vi "2D data.vi"() -> ()   [LabVIEW 2019]
panel:
  out "sorted array":T1(array[cluster])
  out "Array":T1(array[cluster])
  in  "dt 2":u32
  out "XY Graph 3":cluster{"X":dbl, "Y":dbl}[](graph)
  out "Waveform Graph 2":dbl[](graph)
  out "XY Graph 2":cluster{"X":dbl, "Y":dbl}[](graph)
  in  "dt":u32
  in  "index":i32
  in  "stop":bool
  out "XY Graph":cluster{"X":dbl, "Y":dbl}[](graph)
  out "Array 3":cluster{"Array":cluster{"x":dbl, "y":dbl}[]}[](array[cluster])
  out "Array 2":cluster{"x":dbl, "y":dbl}[](array[cluster]) {"x" format="%.3f"; "y" format="%.3f"}
  in  "limit_ptn":dbl
  in  "limit_len":dbl
  out "Waveform Graph":dbl[](graph)
  out "XY 그래프":cluster{"X":dbl, "Y":dbl}[](graph)
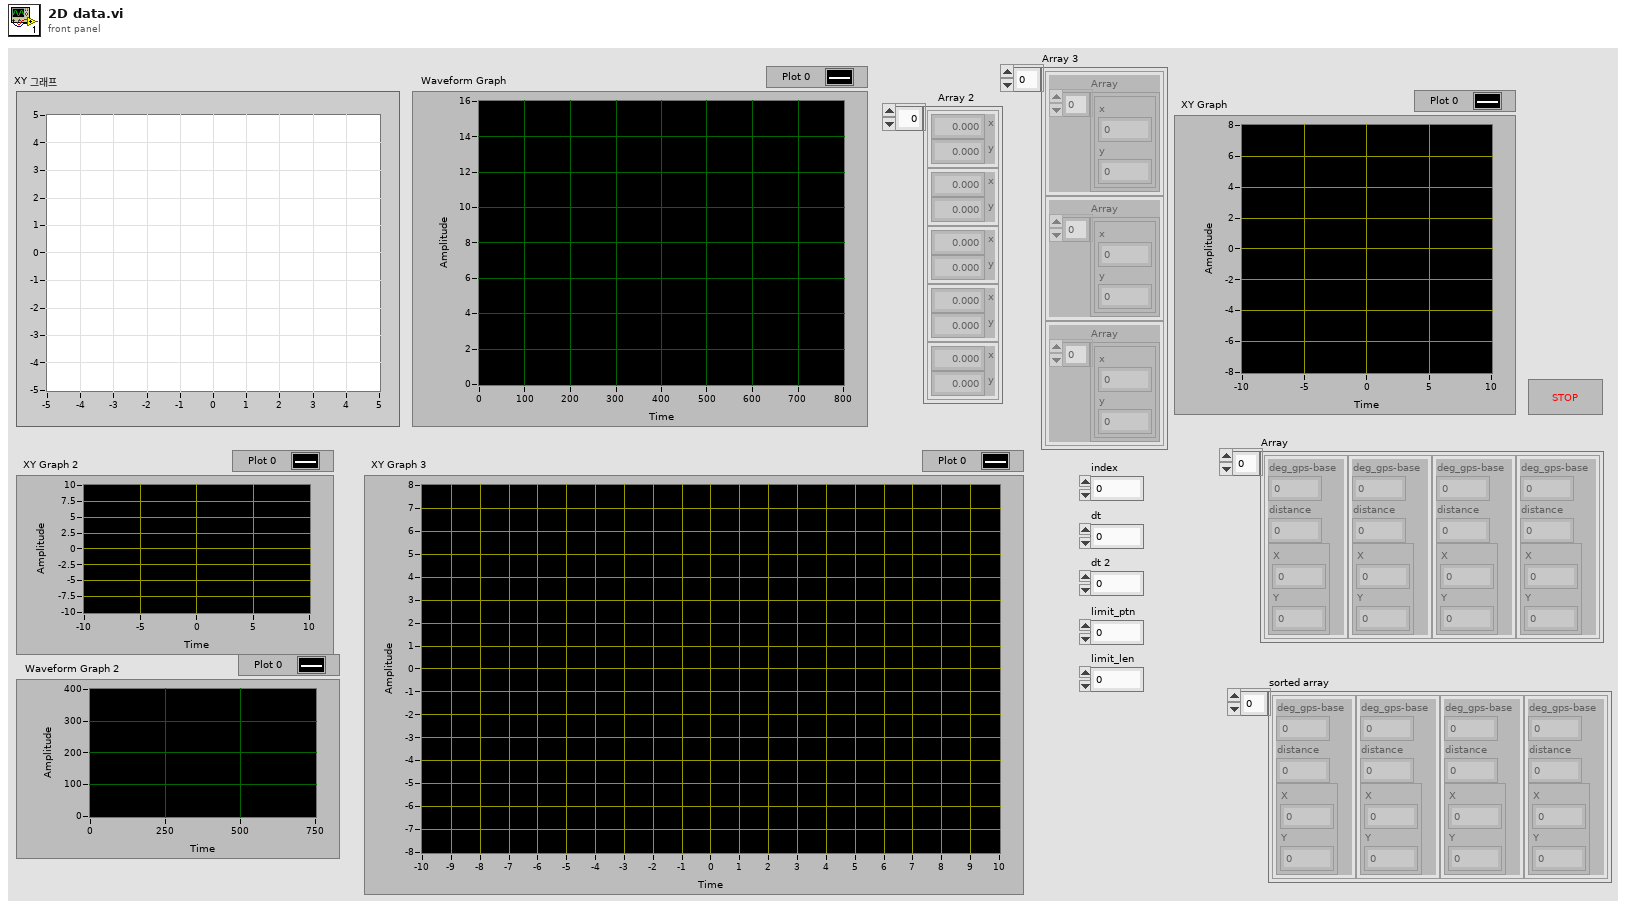
[diagram p1: front panel]
types:
  T1 = cluster{"deg_gps-base":dbl, "distance":dbl, cluster{"X":dbl, "Y":dbl}}[]
  T2 = cluster{"deg_gps-base":dbl, "distance":dbl, "xy":cluster{"X":dbl, "Y":dbl}}
  T3 = cluster{"deg_gps-base":dbl, "distance":dbl, "xy":cluster{"X":dbl, "Y":dbl}}[]
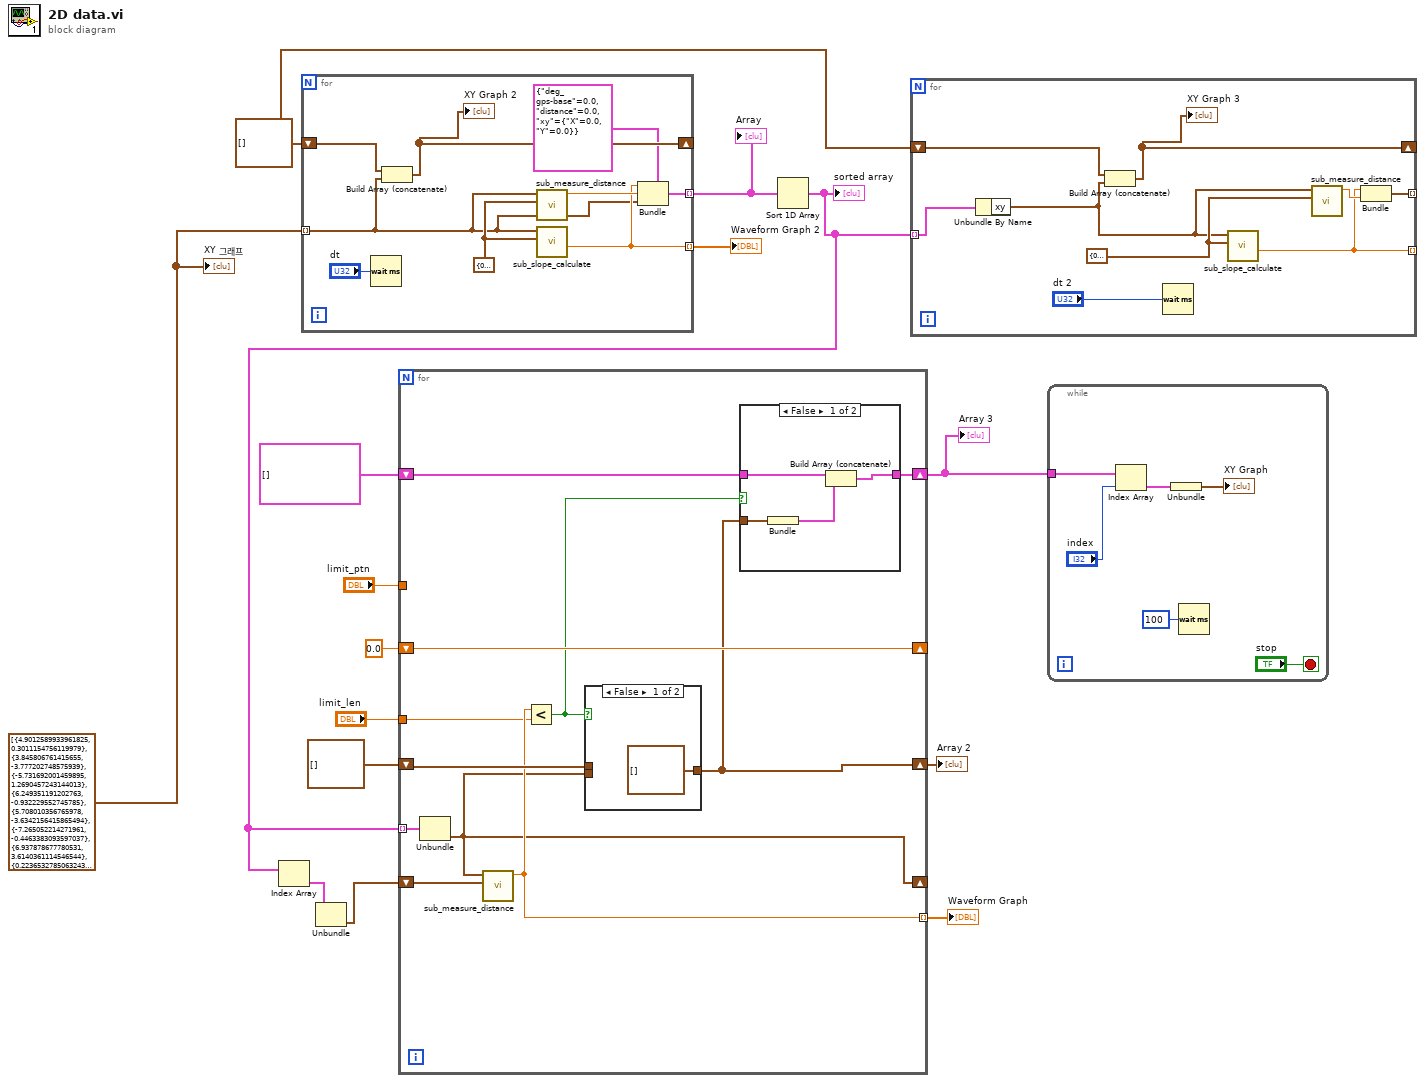
[diagram p0: block diagram]
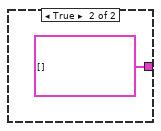
[diagram p2: hidden frame]
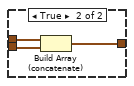
[diagram p3: hidden frame]
diagram:
  w4 = cluster{"X":dbl, "Y":dbl}[] []
  w7 = cluster{"X":dbl, "Y":dbl}[] [{"X"=4.9012589933961825, "Y"=0.3011154756119979}, {"X"=3.845806761415655, "Y"=-3.777202748575939}, {"X"=-5.731692001459895, "Y"=1.2690457243144013}, {"X"=6.249351191202763, "Y"=-0.932229552745785}, {"X"=5.708010356765978, "Y"=-3.6342156415865494}, {"X"=-7.265052214271961, "Y"=-0.4463383093597037}, {"X"=6.937878677780531, "Y"=3.6140361114546544}, {"X"=0.2236532785063243, "Y"=-0.08355102341307699}, {"X"=-0.27698848468565956, "Y"=-0.16663715627537012}, {"X"=-0.2822133509219429, "Y"=-0.16468511487504972}, {"X"=-0.2859435267244487, "Y"=-0.1632233501199644}, {"X"=-0.28971777798992493, "Y"=-0.16059318670659908}, {"X"=-0.2940448834529576, "Y"=-0.15840961623315852}, {"X"=-0.29848859861914145, "Y"=-0.15590099099871388}, {"X"=-0.3029295017509801, "Y"=-0.15383035938625036}, {"X"=-0.30807578671647845, "Y"=-0.15192616509022697}, {"X"=-0.31198972851346785, "Y"=-0.15017147466177655}, {"X"=-0.3163416286007537, "Y"=-0.14740751003331817}, {"X"=-0.32101017207613314, "Y"=-0.14502596982489518}, {"X"=-0.3256611193653853, "Y"=-0.14318832994935127}, {"X"=-0.33034585271792694, "Y"=-0.14118137303506342}, {"X"=-0.3370576037947027, "Y"=-0.1387530962687796}, {"X"=-0.34264737327116335, "Y"=-0.13626936592782707}, {"X"=-0.3452073355688534, "Y"=-0.13316116351794555}, {"X"=-0.34984706268427646, "Y"=-0.13080245690041115}, {"X"=-0.35583414812945, "Y"=-0.1275384609636978}, {"X"=-0.3600731071546751, "Y"=-0.12453255600034033}, {"X"=-0.001185404569007749, "Y"=-0.0003966308205063658}, {"X"=-0.37126244120133567, "Y"=-0.10002224629163652}, {"X"=-0.3684838809764134, "Y"=-0.09486769450429589}, {"X"=-0.36852848189245996, "Y"=-0.08953949147744147}, {"X"=-0.3669884185966218, "Y"=-0.08409370140474674}, {"X"=-0.3637742793807322, "Y"=-0.0789831384602372}, {"X"=-0.3613291353197761, "Y"=-0.07484821954504285}, {"X"=-0.36027625980387135, "Y"=-0.06992865379608967}, {"X"=-0.44303585980691584, "Y"=-0.051334461379728295}, {"X"=-0.43939260085108517, "Y"=-0.04557636248450506}, {"X"=-0.43576159671713005, "Y"=-0.038962556724851855}, {"X"=-0.4316928549636685, "Y"=-0.033619621849704316}, {"X"=-0.42755947741780514, "Y"=-0.0283750466116507}, {"X"=-0.42859886954830667, "Y"=-0.023634117751961833}, {"X"=-0.6725479291533878, "Y"=0.035798505436534504}, {"X"=-0.6768219084672508, "Y"=0.04399052987574099}, {"X"=-0.6817718418184125, "Y"=0.05197324507407022}, {"X"=-0.09026899761251043, "Y"=0.020193020329623453}, {"X"=-0.0896893661121508, "Y"=0.02158425598441085}, {"X"=-0.08952193963087714, "Y"=0.022268471539950586}, {"X"=-0.0892546609486215, "Y"=0.02331668927928274}, {"X"=-0.07805565905243438, "Y"=0.030354185706259997}, {"X"=-0.07791772256148083, "Y"=0.03138197748441136}, {"X"=-0.07754437526468404, "Y"=0.032293495704396255}, {"X"=-0.07738092509395873, "Y"=0.03332048816573892}, {"X"=-0.07697554697222125, "Y"=0.034246571628812124}, {"X"=-0.07679588050516185, "Y"=0.03525113810129967}, {"X"=-0.07659331791069338, "Y"=0.036277074736415234}, {"X"=-0.07638732958398609, "Y"=0.03728238027577482}, {"X"=-0.07397512341025009, "Y"=0.04287109884803828}, {"X"=-0.0736701759708319, "Y"=0.0438835695041625}, {"X"=-0.0731383201458594, "Y"=0.044764367819078804}, {"X"=-0.0726083773719352, "Y"=0.04561892190105601}, {"X"=-0.07205577575029674, "Y"=0.046486854927204405}, {"X"=-0.07171418069777646, "Y"=0.04746658073683699}, {"X"=-0.30349256036447975, "Y"=0.18941311544719558}, {"X"=-0.07241775775620556, "Y"=0.06302117391451487}, {"X"=-0.2622113232445616, "Y"=0.22112037889424854}, {"X"=-0.25329669426595347, "Y"=0.21885691027230578}, {"X"=-0.09164132190783866, "Y"=0.1212677538300429}, {"X"=-0.47795969278638545, "Y"=1.1728498548712636}, {"X"=-0.46467851547189415, "Y"=1.1787123810577524}, {"X"=-0.45634001498452575, "Y"=1.1985658266127575}, {"X"=-0.4477714622363531, "Y"=1.2188531361926747}, {"X"=-0.4381215027443248, "Y"=1.2372169570584841}, {"X"=-0.42844417244887695, "Y"=1.2554034574966715}, {"X"=-0.41821574494214053, "Y"=1.2741179657639596}, {"X"=-0.40855257832630026, "Y"=1.2982317939193033}, {"X"=-0.39994657812166257, "Y"=1.3223407218447039}, {"X"=-0.38933313806268954, "Y"=1.3452954908146608}, {"X"=-0.37866543742498726, "Y"=1.3683210694130759}, {"X"=-0.3683373617066355, "Y"=1.3928704715338736}, {"X"=-0.35666179288220695, "Y"=1.417312462196692}, {"X"=-0.3464174300276499, "Y"=1.4412008974022457}, {"X"=-0.334594909366112, "Y"=1.4693860100825389}, {"X"=-0.32250081681173287, "Y"=1.4971591342124475}, {"X"=-0.31009933090341363, "Y"=1.526317350675558}, {"X"=-0.2978575334569311, "Y"=1.5572704131790833}, {"X"=-0.28460174471109145, "Y"=1.5887094910358541}, {"X"=-0.27027815122515675, "Y"=1.6178287250108745}, {"X"=-0.255080381997715, "Y"=1.645344644358713}, {"X"=-0.24068774355416753, "Y"=1.679339650012112}, {"X"=-0.22553793973565212, "Y"=1.7167483472366583}, {"X"=-0.20853236568394276, "Y"=1.749616601562256}, {"X"=-0.1925175836428063, "Y"=1.789423662101386}, {"X"=-0.1757384256823973, "Y"=1.8356067132527796}, {"X"=-0.15763028421755598, "Y"=1.8783976398775346}, {"X"=-0.13866817212286534, "Y"=1.9227561469255803}, {"X"=-0.11855148061995585, "Y"=1.964676464190177}, {"X"=-0.0980175454142943, "Y"=2.0063571773966262}, {"X"=-0.0762452245746638, "Y"=2.0548359370591025}, {"X"=-0.05341893762434892, "Y"=2.1058225630624925}, {"X"=-0.029492423371756782, "Y"=2.162798926614229}, {"X"=-0.004842739417268302, "Y"=2.219744717388677}, {"X"=0.021733109808708833, "Y"=2.276896280452415}, {"X"=0.04970172896642542, "Y"=2.336221372352746}, {"X"=0.07845218083591374, "Y"=2.396466214621456}, {"X"=0.14265864325553568, "Y"=2.5367418224968206}, {"X"=0.25791276364961613, "Y"=2.823745961722941}, {"X"=0.4003265014221064, "Y"=3.153693024417427}, {"X"=-0.0012014831147085605, "Y"=0.00034487436128279557}, {"X"=0.0012377875979294013, "Y"=-0.00017430393688084778}, {"X"=0.04639406400743008, "Y"=0.0791558799134624}, {"X"=0.24300332766399038, "Y"=0.19167585331550585}, {"X"=0.24014312819302483, "Y"=0.18312639892071392}, {"X"=0.23805466375817233, "Y"=0.17675470874345472}, {"X"=0.23463094212327776, "Y"=0.1708607137359056}, {"X"=0.2322832439149199, "Y"=0.1634028598169623}, {"X"=0.22938017539901892, "Y"=0.15838654499014523}, {"X"=0.22611851588549428, "Y"=0.15117677326144208}, {"X"=0.2227458706393688, "Y"=0.14448019626616504}, {"X"=0.2205770531240713, "Y"=0.13858576274314982}, {"X"=0.21835373612224912, "Y"=0.13315295123073764}, {"X"=0.2154656316353282, "Y"=0.1287461128888521}, {"X"=0.21339293731583509, "Y"=0.12289229757686229}, {"X"=0.21078837067537692, "Y"=0.11887919409223763}, {"X"=0.20887911565298323, "Y"=0.11407679450277194}, {"X"=0.20607850997585403, "Y"=0.10979024422111391}, {"X"=0.20314478914778908, "Y"=0.10624385696171011}, {"X"=0.20184097414595656, "Y"=0.10166720786866974}, {"X"=0.2005907580800803, "Y"=0.09742868044297169}, {"X"=0.1980203433841675, "Y"=0.09411963719658291}, {"X"=2.729292136992012, "Y"=4.636309354535521}, {"X"=-4.581873518186091, "Y"=-0.933494008199846}, {"X"=1.9500741588470802, "Y"=3.31263441614025}, {"X"=2.649775799697403, "Y"=1.6247788384386317}, {"X"=-1.5225966442666026, "Y"=1.9831665389896234}, {"X"=0.21369605927895755, "Y"=1.880144690375888}, {"X"=0.28518527170938746, "Y"=-1.1864566672660417}, {"X"=-0.4894628897939867, "Y"=0.3116346290361832}, {"X"=0.003032126655415368, "Y"=-0.0029780375997491403}, {"X"=0.19986611205371943, "Y"=-7.5538563520398325}, {"X"=-3.486314819830847, "Y"=6.158121566437919}, {"X"=6.107354122634262, "Y"=2.6575337948448157}, {"X"=-3.102921069872052, "Y"=-5.271001146285597}, {"X"=5.5748149068947335, "Y"=-0.8316074818472133}, {"X"=4.9208201278838075, "Y"=1.7440641706983109}, {"X"=0.17247337643341262, "Y"=0.03245280298615732}, {"X"=0.1696371330024223, "Y"=0.031296854581866325}, {"X"=0.16903062835782462, "Y"=0.027481069428953724}, {"X"=0.1678441636080445, "Y"=0.025365315742485833}, {"X"=0.16637140556297375, "Y"=0.023335711066956963}, {"X"=0.16549038973642566, "Y"=0.020457111352435327}, {"X"=0.16455820230675086, "Y"=0.019840880866797528}, {"X"=0.16355135160505668, "Y"=0.017641014374438047}, {"X"=0.16261708964053764, "Y"=0.014361220590233342}, {"X"=0.16171810615316123, "Y"=0.013126943369835676}, {"X"=0.16160845187940687, "Y"=0.011256477297158392}, {"X"=0.15599941991835894, "Y"=0.00042542347786439543}, {"X"=0.1554657184320532, "Y"=-0.0032650256362786022}, {"X"=0.1546615297133665, "Y"=-0.005231990703494369}, {"X"=0.1536518983487234, "Y"=-0.0054915056071692565}, {"X"=0.15276097087023535, "Y"=-0.008549022095135134}, {"X"=0.1517484331234793, "Y"=-0.008741455517757958}, {"X"=0.15086996384425236, "Y"=-0.010715246596974903}, {"X"=0.15024577732585895, "Y"=-0.012319451925650479}, {"X"=0.14928171295419715, "Y"=-0.014661861323197682}, {"X"=0.1489167977985634, "Y"=-0.015774974910337587}, {"X"=0.14791399896350846, "Y"=-0.017956862493855297}, {"X"=0.14693376475094258, "Y"=-0.019711196719495977}, {"X"=0.14589293811695267, "Y"=-0.02335194012503056}, {"X"=0.14549938542039648, "Y"=-0.022638271627642453}, {"X"=0.1445457715006268, "Y"=-0.026749204498238435}, {"X"=0.1436310342800627, "Y"=-0.027553375322080784}, {"X"=0.14261846553712199, "Y"=-0.028813595538161384}, {"X"=0.1421005980970259, "Y"=-0.030082927391919728}, {"X"=0.14169008506375547, "Y"=-0.03307823747761865}, {"X"=0.1407785524831538, "Y"=-0.03473325727235952}, {"X"=0.14049792445394124, "Y"=-0.034826652496825136}, {"X"=0.13938062640994986, "Y"=-0.03812205374281391}, {"X"=0.1386996329763421, "Y"=-0.03870932461601452}, {"X"=0.13740020702170522, "Y"=-0.041393636109824286}, {"X"=0.1366715192368391, "Y"=-0.0420701298963329}, {"X"=0.13611966210438514, "Y"=-0.04300000103009323}, {"X"=0.13456304061514524, "Y"=-0.04612863102680125}, {"X"=0.13412435176580803, "Y"=-0.04663323132061289}, {"X"=0.13321548031702446, "Y"=-0.04770624491515202}, {"X"=0.13301921840476857, "Y"=-0.04825077755834076}, {"X"=0.13225315202414153, "Y"=-0.05031256085391904}, {"X"=0.13163214554167693, "Y"=-0.051230271911193156}, {"X"=0.13103674684671215, "Y"=-0.05273455675200719}, {"X"=0.1302061604170599, "Y"=-0.055394997873877264}, {"X"=0.12138843206985007, "Y"=-0.07271243744795931}, {"X"=0.1205780929457707, "Y"=-0.0745250696179553}, {"X"=0.12023777943807343, "Y"=-0.07554387066997036}, {"X"=0.11940641736415736, "Y"=-0.0773121594075386}, {"X"=0.1190083724126919, "Y"=-0.079284344581273}, {"X"=0.11816660110574537, "Y"=-0.08097664405935613}, {"X"=0.11766043946875705, "Y"=-0.08214786049568765}, {"X"=0.11623652101598524, "Y"=-0.08542326194954407}, {"X"=0.11674060584476939, "Y"=-0.08515797641440404}, {"X"=0.11569744652366608, "Y"=-0.08698657004333157}, {"X"=0.11520452877328761, "Y"=-0.088050647641711}, {"X"=0.11312930964592384, "Y"=-0.09110061360406244}, {"X"=0.11309970397176107, "Y"=-0.09153527714220355}, {"X"=0.11195696687178326, "Y"=-0.09332041614175551}, {"X"=0.11039630593992714, "Y"=-0.09554399842385711}, {"X"=0.1105592363992419, "Y"=-0.09573775507508282}, {"X"=0.10990925202578607, "Y"=-0.0972394920756595}, {"X"=0.1083125701417636, "Y"=-0.10012310996610892}, {"X"=0.1074109559378034, "Y"=-0.10181790876131395}, {"X"=0.10736744916484683, "Y"=-0.10295044128042401}, {"X"=0.10682282567360994, "Y"=-0.10423265522428919}, {"X"=0.10670045487276487, "Y"=-0.10542776166619997}, {"X"=0.10563311410626554, "Y"=-0.10720025748202607}, {"X"=0.10363392728686185, "Y"=-0.11016610919471302}, {"X"=0.1029949423593599, "Y"=-0.11178569608135082}, {"X"=0.10334986872664384, "Y"=-0.1124782962805958}, {"X"=0.10211911023668906, "Y"=-0.11460339141782389}, {"X"=0.10128641403867643, "Y"=-0.11600457892335893}, {"X"=0.1010465383277412, "Y"=-0.11720562952341634}, {"X"=0.10014670362851506, "Y"=-0.11928411567489766}, {"X"=0.09884516278574038, "Y"=-0.12165605736608631}, {"X"=0.09854944602483558, "Y"=-0.12285868584759493}, {"X"=0.09707061217712165, "Y"=-0.12529783019493532}, {"X"=0.09615090678151533, "Y"=-0.1269470977419033}, {"X"=0.09457435243662923, "Y"=-0.12905693263514456}, {"X"=0.09449128674135132, "Y"=-0.13035488763358177}, {"X"=0.09367793739589464, "Y"=-0.13247455055689314}, {"X"=0.09338369059535082, "Y"=-0.13359822727413634}, {"X"=0.09147574883227937, "Y"=-0.13641938966134448}, {"X"=0.09049236429539158, "Y"=-0.1382703674119301}, {"X"=0.08911546167689198, "Y"=-0.14064382137198347}, {"X"=0.08980217302511442, "Y"=-0.14198439956547132}, {"X"=0.08806636250044494, "Y"=-0.14424047904780482}, {"X"=0.08750706041065447, "Y"=-0.14545644323400073}, {"X"=0.08554409842940137, "Y"=-0.14835352952963704}, {"X"=0.08473817761199753, "Y"=-0.14996500843529317}, {"X"=0.08423858827961792, "Y"=-0.15167765242334488}, {"X"=0.08198892401847553, "Y"=-0.15460535675807824}, {"X"=0.08222355680975706, "Y"=-0.15617790082323638}, {"X"=0.08082635570521021, "Y"=-0.15831033675478942}, {"X"=0.07989345221572158, "Y"=-0.16046058330024293}, {"X"=0.07754783575225836, "Y"=-0.16326939599980383}, {"X"=0.07658614667841482, "Y"=-0.16565268526936813}, {"X"=0.07567494859403318, "Y"=-0.16799215652907856}, {"X"=0.07468600223252753, "Y"=-0.17061964591020254}, {"X"=0.05095141617254501, "Y"=-0.1479736570812931}, {"X"=0.05127524789335749, "Y"=-0.14812633612384643}, {"X"=-0.23971296765209224, "Y"=-0.2066638409094029}, {"X"=1.4722460384633376, "Y"=-3.734527368319719}, {"X"=-2.1912542246704536, "Y"=2.8540861909486703}, {"X"=1.8742323048544587, "Y"=3.183800169206595}, {"X"=1.7844117952410417, "Y"=-3.738473056610766}, {"X"=-2.5523798089531446, "Y"=3.853941302205874}, {"X"=3.6175054603020285, "Y"=-3.5529740351830625}, {"X"=-1.7597639864660441, "Y"=-5.264150545143741}, {"X"=-2.9552263755748367, "Y"=5.220022923235761}, {"X"=3.286691716084944, "Y"=5.583176436932528}, {"X"=-1.2604425323685238, "Y"=-6.81110491661202}, {"X"=-2.248440805212299, "Y"=7.124368007616976}, {"X"=2.561335610424748, "Y"=7.661968510328798}, {"X"=0.013085920590032118, "Y"=-0.4945769112911675}, {"X"=-0.27906859118407806, "Y"=-0.1651023437584516}, {"X"=-0.2826166985836709, "Y"=-0.16399196377160233}, {"X"=-0.2869616773770389, "Y"=-0.16142663416226025}, {"X"=-0.29054791102099187, "Y"=-0.15960626993115837}, {"X"=-0.29503960196308593, "Y"=-0.1570818123573312}, {"X"=-0.2998322954542379, "Y"=-0.15494142313352674}, {"X"=-0.30472906443905046, "Y"=-0.15359609300402483}, {"X"=-0.3089143451321374, "Y"=-0.1519209987841797}, {"X"=-0.3132963801071292, "Y"=-0.14859657032303694}, {"X"=-0.3176500148898847, "Y"=-0.14696417264236894}, {"X"=-0.32327718652451126, "Y"=-0.14424930042394093}, {"X"=-0.32781364724239126, "Y"=-0.14200625050201507}, {"X"=-0.3334151423682849, "Y"=-0.14034744507662522}, {"X"=-0.3399047501004513, "Y"=-0.13905870472268103}, {"X"=-0.3436043184487534, "Y"=-0.13589084716553834}, {"X"=-0.34733089163542136, "Y"=-0.1318085798259855}, {"X"=-0.35162256226003075, "Y"=-0.12961148178186532}, {"X"=-0.35692191051120076, "Y"=-0.1267213963663374}, {"X"=-0.3616276198735066, "Y"=-0.12385688129701401}, {"X"=-0.36705871227702547, "Y"=-0.12103781120596918}, {"X"=-0.37254280360963005, "Y"=-0.10386251479083604}, {"X"=-0.36965331014985475, "Y"=-0.09732159470156297}, {"X"=-0.3692382620467948, "Y"=-0.09291753516243602}, {"X"=-0.3675317518758974, "Y"=-0.08834257955840893}, {"X"=-0.365243145833, "Y"=-0.0827507971080274}, {"X"=-0.3627236134028181, "Y"=-0.07792676228358889}, {"X"=-0.36067219417394947, "Y"=-0.07307235010418697}, {"X"=-0.44329589820363263, "Y"=-0.04903821607516491}, {"X"=-0.43713489119076254, "Y"=-0.04305402888975943}, {"X"=-0.43388393682219706, "Y"=-0.037483054406913796}, {"X"=-0.430597413837248, "Y"=-0.031526650578103395}, {"X"=-0.426923420589336, "Y"=-0.026579229716093288}, {"X"=-0.43093302206361084, "Y"=-0.022112903362594794}, {"X"=-0.6754014809486842, "Y"=0.03853685939881598}, {"X"=-0.6783564646789917, "Y"=0.04724941087696129}, {"X"=-0.09018147576304164, "Y"=0.019425857232048514}, {"X"=-0.08945440579688614, "Y"=0.02039538632941347}, {"X"=-0.0892090958587661, "Y"=0.021442940937788375}, {"X"=-0.08918774114899526, "Y"=0.022573143971095798}, {"X"=-0.07756580177106645, "Y"=0.03158494729474193}, {"X"=-0.07741162658180349, "Y"=0.03261042885273693}, {"X"=-0.07701476614556738, "Y"=0.033536931814696}, {"X"=-0.07684423602576869, "Y"=0.03454020685543086}, {"X"=-0.0766607355353628, "Y"=0.03554408005810761}, {"X"=-0.07358334885691208, "Y"=0.043047105256938875}, {"X"=-0.07350209603520613, "Y"=0.04416451492353714}, {"X"=-0.07276639498583365, "Y"=0.04489211245603891}, {"X"=-0.07222250286669421, "Y"=0.04576199383407968}, {"X"=-0.07166821232493865, "Y"=0.046625286510084976}, {"X"=-0.07173717052518366, "Y"=0.0469770248636578}, {"X"=-0.29936861481927335, "Y"=0.18752065209248167}, {"X"=-0.2881723829919772, "Y"=0.18602601345168152}, {"X"=-0.07309913281901172, "Y"=0.061066187707343296}, {"X"=-0.2651661342729049, "Y"=0.21992537651386154}, {"X"=-0.25806687414631296, "Y"=0.2194380344615561}, {"X"=-0.24958224018998745, "Y"=0.2177963908831995}, {"X"=-0.09185762333553107, "Y"=0.1198464727689042}, {"X"=-0.10669222459724777, "Y"=0.22165912841678873}, {"X"=-0.47352297081459477, "Y"=1.1692554238107773}, {"X"=-0.4645677501031146, "Y"=1.1860083760514215}, {"X"=-0.4548110237924447, "Y"=1.2034239413593484}, {"X"=-0.4450448787159056, "Y"=1.2217140084441795}, {"X"=-0.4354979642515731, "Y"=1.2394678638967351}, {"X"=-0.42541950961213143, "Y"=1.257751288348127}, {"X"=-0.4162859580979278, "Y"=1.2800085941471215}, {"X"=-0.4077891645259329, "Y"=1.304497435718155}, {"X"=-0.3979168672241695, "Y"=1.3286952874073508}, {"X"=-0.38736288259283663, "Y"=1.349505834440655}, {"X"=-0.3762746965060186, "Y"=1.3713137324366382}, {"X"=-0.3651700800038398, "Y"=1.396288428359266}, {"X"=-0.3545970184752132, "Y"=1.4222109607890419}, {"X"=-0.34444987491941026, "Y"=1.450410233750439}, {"X"=-0.3329451798473146, "Y"=1.4751432370168123}, {"X"=-0.3194422025248859, "Y"=1.4988371923748254}, {"X"=-0.30765086021354127, "Y"=1.5270677819631544}, {"X"=-0.29492369081800335, "Y"=1.56037303764013}, {"X"=-0.28226627011737554, "Y"=1.5931885490280253}, {"X"=-0.2676424012745098, "Y"=1.6238413123024105}, {"X"=-0.2530384055249634, "Y"=1.6560296277027728}, {"X"=-0.23856639495260729, "Y"=1.6874697442322681}, {"X"=-0.2221763193697196, "Y"=1.7202115954472939}, {"X"=-0.20658949907141605, "Y"=1.7619298450487242}, {"X"=-0.1905985676889359, "Y"=1.8039590311298443}, {"X"=-0.17286448524426382, "Y"=1.8426593370021587}, {"X"=-0.15484100521476835, "Y"=1.8884125146810693}, {"X"=-0.1356102184072145, "Y"=1.9317458732099178}, {"X"=-0.11551242470848723, "Y"=1.967862658377857}, {"X"=-0.09419904798169827, "Y"=2.0067903576007486}, {"X"=-0.07241043111375514, "Y"=2.057476194750724}, {"X"=-0.05020452614241935, "Y"=2.1156544065737237}, {"X"=-0.025439908817034194, "Y"=2.169350838624168}, {"X"=-0.0006054792537042189, "Y"=2.220249917440573}, {"X"=0.05394231834435676, "Y"=2.3543821325969234}, {"X"=0.08387513893575721, "Y"=2.4207973941593104}, {"X"=0.11540740682940795, "Y"=2.487574359280323}, {"X"=0.1477048028989528, "Y"=2.5519791052633214}, {"X"=0.4081328747492611, "Y"=3.1736142832815877}, {"X"=-0.0009573364018852147, "Y"=0.0008037456149961074}, {"X"=0.0010598794394529381, "Y"=-0.0006626881422093846}, {"X"=0.04439114894093455, "Y"=0.07972445293449035}, {"X"=0.045447131233959236, "Y"=0.07941541577428961}, {"X"=0.04652352034983886, "Y"=0.07907986187556304}, {"X"=0.04742620777057602, "Y"=0.07854181890243028}, {"X"=0.24437733678648468, "Y"=0.19275964246995542}, {"X"=0.24158490643859143, "Y"=0.18412168661256892}, {"X"=0.23825538438528715, "Y"=0.176903743067859}, {"X"=0.23518882514902933, "Y"=0.1700919722533057}, {"X"=0.23133205478579727, "Y"=0.16301681026379117}, {"X"=0.22874562957943245, "Y"=0.15666205490899535}, {"X"=0.2259084033897118, "Y"=0.150590980068234}, {"X"=0.22287670343149646, "Y"=0.14473782355524345}, {"X"=0.22097768241790663, "Y"=0.13841757971157712}, {"X"=0.21814029160991066, "Y"=0.13302279194312205}, {"X"=0.2153911966821918, "Y"=0.12838300078987624}, {"X"=0.21332587822874813, "Y"=0.12300866708461371}, {"X"=0.21114403371161689, "Y"=0.1182463404422631}, {"X"=0.20850468241850678, "Y"=0.11475973775483124}, {"X"=0.2057381123677105, "Y"=0.10989718658533223}, {"X"=0.20360643016333815, "Y"=0.10535646205212904}, {"X"=0.20195175575741012, "Y"=0.101446973077068}, {"X"=0.20031277122013877, "Y"=0.097428723619415}, {"X"=0.19835502076690129, "Y"=0.09282395023140401}, {"X"=0.19587672532844022, "Y"=0.08984741774033789}, {"X"=0.1948676521099114, "Y"=0.08599766369600136}, {"X"=0.19296875339069683, "Y"=0.08284358885780137}, {"X"=0.1913341430043682, "Y"=0.07833778284317205}, {"X"=0.18978478747891206, "Y"=0.07481800880526149}, {"X"=0.1886049874425679, "Y"=0.07163254296609053}, {"X"=0.18710332316129352, "Y"=0.0685048097727493}, {"X"=0.18512147871699317, "Y"=0.06589604022726896}, {"X"=0.18406003677848523, "Y"=0.06208836735736147}, {"X"=0.18235862266877167, "Y"=0.06007772247970582}, {"X"=0.1805683621457713, "Y"=0.056662413397185814}, {"X"=0.1795740759467218, "Y"=0.05393886583791857}, {"X"=0.17856831591639727, "Y"=0.05115094379170087}, {"X"=0.17729284466571532, "Y"=0.04828363832954744}, {"X"=0.176412236284399, "Y"=0.04475179202151994}, {"X"=0.17514266322228852, "Y"=0.04260410801089521}, {"X"=0.17413077548639438, "Y"=0.03925204489586392}, {"X"=0.17203016389920311, "Y"=0.03343927643973949}, {"X"=0.16982184650315332, "Y"=0.03027854769072372}, {"X"=0.1688549356634863, "Y"=0.028540728828813967}, {"X"=0.16776731804757072, "Y"=0.02586869720579792}, {"X"=0.1664281788529168, "Y"=0.022927304326970974}, {"X"=0.16525339452438775, "Y"=0.02033631230501384}, {"X"=0.16447160698406382, "Y"=0.018421196923100718}, {"X"=0.16332665914856592, "Y"=0.017391518374430967}, {"X"=0.16260528597385776, "Y"=0.014494256564582492}, {"X"=0.16170369066696158, "Y"=0.013303342613178181}, {"X"=0.16158350947555758, "Y"=0.011609025177093408}, {"X"=0.15599941991835894, "Y"=0.00042542347786439543}, {"X"=0.15524445224591968, "Y"=-0.0013124583286203261}, {"X"=0.15445946474998923, "Y"=-0.0035388909487062184}, {"X"=0.15365039505939593, "Y"=-0.0055334074575766135}, {"X"=0.15283753764000332, "Y"=-0.0070489068755775226}, {"X"=0.15167455633226773, "Y"=-0.009941275642981725}, {"X"=0.15079340488049622, "Y"=-0.011743574606853987}, {"X"=0.15022541855219693, "Y"=-0.012565274402783537}, {"X"=0.14930942975507683, "Y"=-0.014376862878033593}, {"X"=0.14886880631303165, "Y"=-0.01622162158765475}, {"X"=0.14795762617913108, "Y"=-0.01759377320066718}, {"X"=0.14675042918614536, "Y"=-0.021032689644506556}, {"X"=0.14625548676055974, "Y"=-0.020961753085840428}, {"X"=0.14539287048077043, "Y"=-0.023312565567991776}, {"X"=0.1448426615709472, "Y"=-0.02509189887282462}, {"X"=0.14409183598505562, "Y"=-0.02780477121746971}, {"X"=0.14273621584208732, "Y"=-0.029486186377371028}, {"X"=0.14225456295943165, "Y"=-0.029346240256992055}, {"X"=0.142042475653038, "Y"=-0.031530701076190944}, {"X"=0.14093806349908553, "Y"=-0.03408023264485936}, {"X"=0.14055472132779298, "Y"=-0.03459671678738397}, {"X"=0.13951490053558194, "Y"=-0.03762768300794885}, {"X"=0.13903215001469754, "Y"=-0.03749748341276564}, {"X"=0.13778903501979314, "Y"=-0.04008031721823348}, {"X"=0.13689894222965154, "Y"=-0.041324080345514394}, {"X"=0.13573923804932692, "Y"=-0.04418621678519397}, {"X"=0.13540716217248813, "Y"=-0.04358856423872542}, {"X"=0.134263637735103, "Y"=-0.04623067793291624}, {"X"=0.13313724286218406, "Y"=-0.04792415427585368}, {"X"=0.13212926820377308, "Y"=-0.05063700705941656}, {"X"=0.13186512279042326, "Y"=-0.05132094495882359}, {"X"=0.13107984634714606, "Y"=-0.052627334927854534}, {"X"=0.13035008938407125, "Y"=-0.054409711426956095}, {"X"=0.1306549971379065, "Y"=-0.05432790924463825}, {"X"=0.12168485425615991, "Y"=-0.07221527708634178}, {"X"=0.12094246285197544, "Y"=-0.0739322877997059}, {"X"=0.11984064575492662, "Y"=-0.07570523182080739}, {"X"=0.119027908188787, "Y"=-0.07743614835593061}, {"X"=0.11915277499230591, "Y"=-0.07770250132159788}, {"X"=0.118994210660949, "Y"=-0.07885391765269299}, {"X"=0.11796037667100584, "Y"=-0.08083532356361554}, {"X"=0.1175034087044206, "Y"=-0.0823723190328031}, {"X"=0.11729894392436713, "Y"=-0.08395844361485136}, {"X"=0.11552130028693207, "Y"=-0.08680483385167248}, {"X"=0.11536449740531828, "Y"=-0.08742765717104807}, {"X"=0.1148433845744308, "Y"=-0.08852116707030803}, {"X"=0.11362450128096858, "Y"=-0.09048223697859802}, {"X"=0.11242266009383559, "Y"=-0.09236555363026795}, {"X"=0.11186648656668836, "Y"=-0.09303837478817507}, {"X"=0.11026592543564984, "Y"=-0.09569443916874015}, {"X"=0.11027154673692342, "Y"=-0.09606897772041978}, {"X"=0.10929718100728303, "Y"=-0.09792695606349258}, {"X"=0.10912806648455785, "Y"=-0.0992336389806497}, {"X"=0.10891818218537794, "Y"=-0.10057281983435096}, {"X"=0.1068890156447301, "Y"=-0.10344709195767972}, {"X"=0.10710667857574158, "Y"=-0.10394095393285929}, {"X"=0.10658538756575843, "Y"=-0.10554409105893645}, {"X"=0.10501508510290937, "Y"=-0.10815449320684141}, {"X"=0.10527458142551772, "Y"=-0.10859937847742057}, {"X"=0.10393628005488878, "Y"=-0.11091099895119387}, {"X"=0.10230253545180715, "Y"=-0.11343171399627064}, {"X"=0.10180619862916933, "Y"=-0.11488145159545173}, {"X"=0.10147609041527338, "Y"=-0.11583869420030278}, {"X"=0.10079059504061141, "Y"=-0.11742579976887312}, {"X"=0.10047162779569585, "Y"=-0.11901056469105235}, {"X"=0.09963927703565825, "Y"=-0.12100651623698346}, {"X"=0.09851593785161007, "Y"=-0.12288555647112358}, {"X"=0.09783599468901896, "Y"=-0.12438320080786736}, {"X"=0.0958043551712464, "Y"=-0.127208836289865}, {"X"=0.09534693171420972, "Y"=-0.1284872079729567}, {"X"=0.09374321691206747, "Y"=-0.13089388558285323}, {"X"=0.09320770090503276, "Y"=-0.1328058243903405}, {"X"=0.09272676939332979, "Y"=-0.13405501198342507}, {"X"=0.09128965076541125, "Y"=-0.13654399350806043}, {"X"=0.09079380784647519, "Y"=-0.1380726147964807}, {"X"=0.0907204764918706, "Y"=-0.13961391458263733}, {"X"=0.0886610651888955, "Y"=-0.14240533002514486}, {"X"=0.08734619323622593, "Y"=-0.14438561225807742}, {"X"=0.08647352502873291, "Y"=-0.14607324179706938}, {"X"=0.0857867267024921, "Y"=-0.14821335979483066}, {"X"=0.0846563717884342, "Y"=-0.15001120363365664}, {"X"=0.0832855732379634, "Y"=-0.15220303311834438}, {"X"=0.0833769335146265, "Y"=-0.15386125879407575}, {"X"=0.08222355680975706, "Y"=-0.15617790082323638}, {"X"=0.08112841538175991, "Y"=-0.15815575461438203}, {"X"=0.07919255253468861, "Y"=-0.16080765567298275}, {"X"=0.07881237896592223, "Y"=-0.1629405073078265}, {"X"=0.07667648480673822, "Y"=-0.1656108893692744}, {"X"=0.07594972369241286, "Y"=-0.16786810885646544}, {"X"=0.07509655139650827, "Y"=-0.17016611874386625}, {"X"=0.05119221555651464, "Y"=-0.14762594476044966}, {"X"=0.04901513463609905, "Y"=-0.1480996845931992}, {"X"=-0.2396200747724744, "Y"=-0.20715400615492277}, {"X"=-0.23690175482196324, "Y"=-0.19955605994876333}, {"X"=-0.2350644565709765, "Y"=-0.1923766195695088}, {"X"=-0.23484795236703623, "Y"=-0.18827490344974365}, {"X"=-0.23782059136117903, "Y"=-0.1865380090614755}, {"X"=-0.24173348003536269, "Y"=-0.18433915652946045}, {"X"=-0.2455807027502072, "Y"=-0.18213506234856144}, {"X"=-0.248579745066811, "Y"=-0.18143365961838293}, {"X"=-0.2522135840707145, "Y"=-0.17938382873103315}, {"X"=-0.25583433435006864, "Y"=-0.1772719827487054}, {"X"=-0.259600442106301, "Y"=-0.17530879315714046}, {"X"=-0.26317399515511175, "Y"=-0.17264706998410725}, {"X"=-0.26684295091611154, "Y"=-0.1711252159863697}, {"X"=-0.27020415228889444, "Y"=-0.16956036118692347}, {"X"=-0.2746720680620595, "Y"=-0.16708532259450967}, {"X"=-0.2784024904998144, "Y"=-0.16573488855247337}, {"X"=-0.28279541788590323, "Y"=-0.16368357927030236}, {"X"=-0.2865646128882119, "Y"=-0.16213045716406657}, {"X"=-0.29046081609335045, "Y"=-0.15976471548619509}, {"X"=-0.29512523291309634, "Y"=-0.15692086986118398}, {"X"=-0.2994086438753615, "Y"=-0.1557585117183551}, {"X"=-0.3043801493597151, "Y"=-0.1537326402419394}, {"X"=-0.3092037922765022, "Y"=-0.15133101909995075}, {"X"=-0.3128492134344373, "Y"=-0.1495357219979692}, {"X"=-0.3177701433534504, "Y"=-0.14670424667720966}, {"X"=-0.32284301579863434, "Y"=-0.14521841188376478}, {"X"=-0.32803932698332067, "Y"=-0.14274194356365624}, {"X"=-0.3328012241862807, "Y"=-0.14051657439644952}, {"X"=-0.3379662853306548, "Y"=-0.13719093439363397}, {"X"=-0.34262626940938057, "Y"=-0.13496407674122243}, {"X"=-0.3471869041611224, "Y"=-0.13218738055887042}, {"X"=-0.3513526553029703, "Y"=-0.12962083787552126}, {"X"=-0.35689305145725775, "Y"=-0.12605395599316657}, {"X"=-0.36142484856398677, "Y"=-0.12367731740500847}, {"X"=-0.36702569068587315, "Y"=-0.1211379064395525}, {"X"=-0.3723585435351147, "Y"=-0.10359230210979997}, {"X"=-0.3694401078263613, "Y"=-0.09812782087281144}, {"X"=-0.36926358764334793, "Y"=-0.0928168375929902}, {"X"=-0.3675798806098077, "Y"=-0.0881421089541176}, {"X"=-0.36535564015722183, "Y"=-0.08225269725247075}, {"X"=-0.3637863227148593, "Y"=-0.07774002447645778}, {"X"=-0.3618310260789739, "Y"=-0.07238306823171387}, {"X"=-0.44307407926156234, "Y"=-0.04876907612943626}, {"X"=-0.4373954189557977, "Y"=-0.04295925367696932}, {"X"=-0.4339043161205179, "Y"=-0.0372464018662975}, {"X"=-0.43058880026547025, "Y"=-0.031644076632806946}, {"X"=-0.42693065307469574, "Y"=-0.026462803426957823}, {"X"=-0.43121246199021723, "Y"=-0.021537760429893704}, {"X"=-0.6756510749919026, "Y"=0.038551100662451904}, {"X"=-0.6788809447284851, "Y"=0.04691388797104268}, {"X"=-0.08994763459045625, "Y"=0.01932415668487915}, {"X"=-0.08922174119941413, "Y"=0.02029115317927417}, {"X"=-0.08921494019648682, "Y"=0.021418612133779345}, {"X"=-0.0892000396228427, "Y"=0.022524496249268035}, {"X"=-0.08916498969054801, "Y"=0.02365728457546354}, {"X"=-0.07793920096814108, "Y"=0.030651973059620762}, {"X"=-0.07757441234488842, "Y"=0.0315637933294657}, {"X"=-0.07719895664989138, "Y"=0.032471273337647114}, {"X"=-0.07703304624835042, "Y"=0.03349492178972068}, {"X"=-0.07317510493127444, "Y"=0.04275472509906919}, {"X"=-0.07329981037407506, "Y"=0.04401576761939565}, {"X"=-0.07277863470442178, "Y"=0.044872266831087707}, {"X"=-0.07223497982884998, "Y"=0.04574229650034679}, {"X"=-0.07169363181270566, "Y"=0.04658619063096059}, {"X"=-0.3017045533722128, "Y"=0.1894424054283349}, {"X"=-0.07202308421869473, "Y"=0.06309308868352226}, {"X"=-0.2690435680809424, "Y"=0.22190565782393956}, {"X"=-0.0892378973530921, "Y"=0.13129417418910483}, {"X"=-0.10692165492568916, "Y"=0.22182610803949984}, {"X"=-0.47301653213948536, "Y"=1.168921023988676}, {"X"=-0.4641531815960967, "Y"=1.1859022194153366}, {"X"=-0.4542428441410986, "Y"=1.2039057276409169}, {"X"=-0.4451304478139091, "Y"=1.2219489082727593}, {"X"=-0.43632669491618126, "Y"=1.2418265087376423}, {"X"=-0.4271574572846804, "Y"=1.264025145788677}, {"X"=-0.4170956881575855, "Y"=1.2836885328693834}, {"X"=-0.4066473929133761, "Y"=1.3045919468695009}, {"X"=-0.39734308659370937, "Y"=1.326779360532935}, {"X"=-0.38621372095752626, "Y"=1.3482749021413036}, {"X"=-0.37572476756859025, "Y"=1.3722421293399822}, {"X"=-0.36491566554975075, "Y"=1.3968717262284258}, {"X"=-0.3533730743148532, "Y"=1.422257965472252}, {"X"=-0.34433434586526995, "Y"=1.449923763774336}, {"X"=-0.33265283426452735, "Y"=1.475721740151502}, {"X"=-0.3191895800383244, "Y"=1.499657819135738}, {"X"=-0.3073330204416971, "Y"=1.527641802598431}, {"X"=-0.29463724329979, "Y"=1.5611903975366683}, {"X"=-0.2814407578046291, "Y"=1.5935884545096188}, {"X"=-0.2671995573054481, "Y"=1.623914240061886}, {"X"=-0.25258678409773605, "Y"=1.6560985716433558}, {"X"=-0.23771570911810116, "Y"=1.6880947260561174}, {"X"=-0.22180306264661753, "Y"=1.7210159685199264}, {"X"=-0.20661861258594136, "Y"=1.7621781440686013}, {"X"=-0.19010660709729582, "Y"=1.8040109417456298}, {"X"=-0.17289747398629612, "Y"=1.8484314197419276}, {"X"=-0.1548147104914289, "Y"=1.8944347357234177}, {"X"=-0.13506597228706327, "Y"=1.9315333923155846}, {"X"=-0.11420578696519602, "Y"=1.9731977316588576}, {"X"=-0.09417620861819202, "Y"=2.018053741660589}, {"X"=-0.07146137598458878, "Y"=2.062512384021582}, {"X"=-0.04847364382006142, "Y"=2.1156947720204835}, {"X"=-0.024819675528223856, "Y"=2.166857859599165}, {"X"=0.02762135424590735, "Y"=2.301834281782601}, {"X"=0.05533781739085846, "Y"=2.35910105516199}, {"X"=0.08510753646023429, "Y"=2.4182528341217076}, {"X"=0.1166938181505489, "Y"=2.48601269411591}, {"X"=0.1497779366163058, "Y"=2.5516078401084603}, {"X"=-0.0008361599002088121, "Y"=0.0009291590936340178}, {"X"=0.0008989379186363499, "Y"=-0.0008685681426564916}, {"X"=0.0465666448016446, "Y"=0.07905447547051}, {"X"=0.04777077556361442, "Y"=0.07891777684432563}, {"X"=0.24385395292664044, "Y"=0.19180800854513824}, {"X"=0.24163669702304738, "Y"=0.18364083601364922}, {"X"=0.23686689855275322, "Y"=0.17667575490145707}, {"X"=0.23367855846572183, "Y"=0.16919391630133224}, {"X"=0.23058589240328395, "Y"=0.16277348901028438}, {"X"=0.22855206563366767, "Y"=0.15561556250768646}, {"X"=0.2249535047532159, "Y"=0.15022040706656625}, {"X"=0.22266703578951008, "Y"=0.1446016637964897}, {"X"=0.22091652904874898, "Y"=0.13804396833274987}, {"X"=0.21746378013292533, "Y"=0.13269162306000598}, {"X"=0.21509521998515851, "Y"=0.12741289706908115}, {"X"=0.21309067180954944, "Y"=0.12341567196979034}, {"X"=0.21084232834750297, "Y"=0.11724792141869192}, {"X"=0.20772013811412618, "Y"=0.11359096232468649}, {"X"=0.2053376987661949, "Y"=0.11011552781239982}, {"X"=0.2038644003106139, "Y"=0.1048564198606541}, {"X"=0.2016453859948876, "Y"=0.10149975766952744}, {"X"=0.19977053233099068, "Y"=0.09682837606916997}, {"X"=0.1977503544995506, "Y"=0.09293571592935658}, {"X"=0.19633963342506547, "Y"=0.08883129148284918}, {"X"=0.19452702140588715, "Y"=0.08553062576032934}, {"X"=0.19300167880145555, "Y"=0.08148988881953265}, {"X"=0.1913127725736825, "Y"=0.0783899582227879}, {"X"=0.18966211279740813, "Y"=0.07512844314388023}, {"X"=0.18842974475173135, "Y"=0.07138964415653973}, {"X"=0.18687488461370763, "Y"=0.06767082089507605}, {"X"=0.18516446615660864, "Y"=0.06426601335805829}, {"X"=0.18412765515980828, "Y"=0.06188755210339743}, {"X"=0.1823200027822165, "Y"=0.05858042834849}, {"X"=0.18021416202783572, "Y"=0.05611967840788973}, {"X"=0.17945173641624465, "Y"=0.05347557196697065}, {"X"=0.17873475052815024, "Y"=0.05056630749461442}, {"X"=0.1774108164250047, "Y"=0.04784835122983117}, {"X"=0.17636331470428127, "Y"=0.0449442012557644}, {"X"=0.17555863041501835, "Y"=0.041945408411445936}, {"X"=0.17401224450574754, "Y"=0.03977422233145406}, {"X"=0.172324125547516, "Y"=0.03188978291371621}, {"X"=0.1699119114015449, "Y"=0.02976898325226366}, {"X"=0.16879880992801463, "Y"=0.027348889682873582}, {"X"=0.167458534933831, "Y"=0.02456016241426154}, {"X"=0.16603365752676053, "Y"=0.0239350593959239}, {"X"=0.1652086343348824, "Y"=0.020696790601518914}, {"X"=0.16438966395333496, "Y"=0.01913866205641355}, {"X"=0.1633502213142389, "Y"=0.01716880009171208}, {"X"=0.16230394676222198, "Y"=0.015047553469113064}, {"X"=0.16157715370109765, "Y"=0.011697153579049376}, {"X"=0.16193976444853678, "Y"=0.004417317098921966}, {"X"=0.15599994779262286, "Y"=0.00012762718731472447}, {"X"=0.15524251834093566, "Y"=-0.0015241388270924772}, {"X"=0.15445751161035173, "Y"=-0.003623134987556989}, {"X"=0.1533975211038901, "Y"=-0.005608076246057275}, {"X"=0.1525897165775659, "Y"=-0.0069957769245535435}, {"X"=0.15210494742894617, "Y"=-0.010969729606399692}, {"X"=0.15121154000135142, "Y"=-0.012772340052617216}, {"X"=0.15021854291410802, "Y"=-0.01264720778521032}, {"X"=0.14924937049625028, "Y"=-0.014987508347721185}, {"X"=0.1486634486112401, "Y"=-0.01800670838918592}, {"X"=0.1484299199927914, "Y"=-0.017855219151092453}, {"X"=0.14729672415359873, "Y"=-0.020742168488820958}, {"X"=0.14603653718240625, "Y"=-0.022436405856813873}, {"X"=0.14518389643478394, "Y"=-0.024580453942389554}, {"X"=0.14493740425068413, "Y"=-0.024538721422962744}, {"X"=0.14374705506957527, "Y"=-0.028267192269917675}, {"X"=0.14306900687464114, "Y"=-0.029107718424910767}, {"X"=0.1420596518545975, "Y"=-0.03145322423775578}, {"X"=0.14131037040819122, "Y"=-0.0335997279021689}, {"X"=0.14100286425508496, "Y"=-0.033811126450653546}, {"X"=0.14055472132779298, "Y"=-0.03459671678738397}, {"X"=0.13964544246171245, "Y"=-0.036155399315628535}, {"X"=0.13892937463134905, "Y"=-0.03787649488194837}, {"X"=0.13838916513321606, "Y"=-0.03980501191723798}, {"X"=0.13745652109003348, "Y"=-0.04120624721841558}, {"X"=0.13616648683466606, "Y"=-0.042851491958912115}, {"X"=0.13498544569806945, "Y"=-0.04643804420616303}, {"X"=0.13439866010991341, "Y"=-0.04660539304265091}, {"X"=0.13330688182623304, "Y"=-0.048190639731868413}, {"X"=0.13271396157041337, "Y"=-0.04908415634689917}, {"X"=0.13132241878742107, "Y"=-0.052019081343495484}, {"X"=0.13081993433030611, "Y"=-0.05327013498963934}, {"X"=0.13015637732883698, "Y"=-0.0548714856791158}, {"X"=0.13049143749136893, "Y"=-0.0547196010716101}, {"X"=0.12170454339289881, "Y"=-0.07218209000524999}, {"X"=0.12047636308563114, "Y"=-0.07468941315647867}, {"X"=0.12050484141055236, "Y"=-0.07511712984810871}, {"X"=0.11971995418467125, "Y"=-0.07636185284564681}, {"X"=0.11887655587664353, "Y"=-0.07812443256054566}, {"X"=0.11825796775455098, "Y"=-0.07995383394536862}, {"X"=0.11792315730308468, "Y"=-0.08133075354176884}, {"X"=0.11831715906367157, "Y"=-0.08207953381386764}, {"X"=0.11720333186871722, "Y"=-0.08451999171125926}, {"X"=0.11653124531665122, "Y"=-0.08544424418853766}, {"X"=0.1150298666877034, "Y"=-0.08786746991810555}, {"X"=0.1147950866881663, "Y"=-0.08858379125018517}, {"X"=0.11396912515631161, "Y"=-0.09004777071701987}, {"X"=0.11279955040895906, "Y"=-0.09190490426270354}, {"X"=0.11186648656668836, "Y"=-0.09303837478817507}, {"X"=0.11132897177033267, "Y"=-0.09445559827008917}, {"X"=0.1105592363992419, "Y"=-0.09573775507508282}, {"X"=0.10998876910781014, "Y"=-0.09714954024671876}, {"X"=0.108476251131574, "Y"=-0.09994574998687883}, {"X"=0.10750891707495636, "Y"=-0.10207788815101022}, {"X"=0.10771648999358562, "Y"=-0.10294735442672517}, {"X"=0.10608109545647126, "Y"=-0.10498744537684034}, {"X"=0.10560220866839523, "Y"=-0.1065278063434928}, {"X"=0.10442792853860451, "Y"=-0.10837461760548966}, {"X"=0.10500772163375173, "Y"=-0.10885743381730302}, {"X"=0.10371272608517342, "Y"=-0.11146180039808164}, {"X"=0.10271760062098294, "Y"=-0.11339353827563652}, {"X"=0.10104275911897574, "Y"=-0.1168786157927302}, {"X"=0.10082680950326103, "Y"=-0.11805302615940481}, {"X"=0.09864249711259589, "Y"=-0.12053099295779285}, {"X"=0.0990772183451178, "Y"=-0.12146714496107107}, {"X"=0.09710200950199613, "Y"=-0.12400584563105989}, {"X"=0.09710477824969148, "Y"=-0.1252713536331361}, {"X"=0.0968763345442604, "Y"=-0.12639437608243706}, {"X"=0.09528521835605575, "Y"=-0.12884405171694494}, {"X"=0.0007305887079749594, "Y"=-0.0010142682780110398}, {"X"=0.0933163212107787, "Y"=-0.13272952458171008}, {"X"=0.09253918384438674, "Y"=-0.1344881480035129}, {"X"=0.09162450484830857, "Y"=-0.13631952395494298}, {"X"=0.08994841744778657, "Y"=-0.1389227562303553}, {"X"=0.08907710371120167, "Y"=-0.14066811861407624}, {"X"=0.08873872205648049, "Y"=-0.1423569517367617}, {"X"=0.0874755950039833, "Y"=-0.14459951686883013}, {"X"=0.08640132899518825, "Y"=-0.14640631935768772}, {"X"=0.08538221896983127, "Y"=-0.14844675538316013}, {"X"=0.0853521811529162, "Y"=-0.14990415328615742}, {"X"=0.08419422631358477, "Y"=-0.15198814018026824}, {"X"=0.08315969225274583, "Y"=-0.15426285387101007}, {"X"=0.07886120294249328, "Y"=-0.1601348202935979}, {"X"=0.07762838261493195, "Y"=-0.16378460462628877}, {"X"=0.07658614667841482, "Y"=-0.16565268526936813}, {"X"=0.05094239423237216, "Y"=-0.14638945477688473}, {"X"=0.049739117881955695, "Y"=-0.14838554563138862}] ("XY 그래프")
  n1 = for {
    tunnel: w7 -> [w17] mode=indexing
    shift-right: [w22] -> _
    shift-left: w4 -> [w24]
    tunnel: [w18] -> w6 mode=indexing
    tunnel: [w20] -> w5 mode=indexing
    w21 = cluster{"x":dbl, "y":dbl} {"x"=0.0, "y"=0.0} ("pt 2")
    n2 = Wait (ms)(milliseconds to wait="dt") -> ()  [unwired: 1 out]
    n3 = Build Array (concatenate)(w24, w17) -> (w22:cluster{"X":dbl, "Y":dbl}[])
    "XY Graph 2" <- w22
    n4 = call "sub_measure_distance.vi"("pt 2"=w21, "pt 1"=w17) -> ("distance"=w19:dbl)  [unwired: 9 in]
    n5 = call "sub_slope_calculate.vi"("point n+1"=w21, "point n"=w17) -> ("deg_gps-base"=w18:dbl)  [unwired: 7 in, 2 out]
    n6 = Bundle(cluster=T2 {"deg_gps-base"=0.0, "distance"=0.0, "xy"={"X"=0.0, "Y"=0.0}}, "deg_gps-base"=w18, "distance"=w19, "xy"=w17) -> (w20:T2)
  }
  "Waveform Graph 2" <- w6
  "Array" <- w5
  n7 = Sort 1D Array(array=w5) -> (sorted array=w3:T3)
  "sorted array" <- w3
  n8 = Index Array(array=w3) -> (element=w2:T2)  [unwired: 1 in]
  n9 = Unbundle(w2) -> ("xy"=w1:cluster{"X":dbl, "Y":dbl})  [unwired: 2 out]
  n10 = for {
    shift-right: [w25] -> _
    shift-left: w1 -> [w35]
    tunnel: [w28] -> w15 mode=indexing
    shift-right: [w30] -> w8
    shift-left: cluster{"Array":cluster{"x":dbl, "y":dbl}[]}[] [] ("Array") -> [w31]
    shift-right: [w33] -> _
    shift-left: 0.0 -> [w33]
    tunnel: "limit_len" -> [w27]
    tunnel: "limit_ptn" -> [_]
    shift-right: [w32] -> w9
    shift-left: cluster{"x":dbl, "y":dbl}[] [] ("Array") -> [w34]
    tunnel: w3 -> [w26] mode=indexing
    n11 = Unbundle(w26) -> ("xy"=w25:cluster{"X":dbl, "Y":dbl})  [unwired: 2 out]
    n12 = call "sub_measure_distance.vi"("pt 2"=w35, "pt 1"=w25) -> ("distance"=w28:dbl)  [unwired: 9 in]
    n13 = Less?(x=w28, y=w27) -> (x < y?=w29:bool)
    n14 = case shown="False" w29 {
      tunnel: w34 -> [_ w44]
      tunnel: w25 -> [_ w43]
      tunnel: [cluster{"x":dbl, "y":dbl}[] [] w42] -> w32
      frame False {
      }
      frame True {
        n15 = Build Array (concatenate)(w44, w43) -> (w42:cluster{"X":dbl, "Y":dbl}[])
      }
    }
    n16 = case shown="False" w29 {
      tunnel: w32 -> [w39 _]
      tunnel: w31 -> [w37 _]
      tunnel: [w36 cluster{"Array":cluster{"x":dbl, "y":dbl}[]}[] []] -> w30
      frame False {
        n17 = Bundle(w39) -> (w38:cluster{cluster{"X":dbl, "Y":dbl}[]})  [unwired: 1 in]
        n18 = Build Array (concatenate)(w37, w38) -> (w36:cluster{"Array":cluster{"X":dbl, "Y":dbl}[]}[])
      }
      frame True {
      }
    }
  }
  "Waveform Graph" <- w15
  "Array 2" <- w9
  "Array 3" <- w8
  n19 = for {
    tunnel: w3 -> [w46] mode=indexing
    shift-right: [w51] -> _
    shift-left: w4 -> [w53]
    tunnel: [w47] -> _ mode=indexing
    tunnel: [w49] -> _ mode=indexing
    w50 = cluster{"x":dbl, "y":dbl} {"x"=0.0, "y"=0.0} ("pt 2")
    n20 = Unbundle By Name(w46) -> ("xy"=w45:cluster{"X":dbl, "Y":dbl})
    n21 = Build Array (concatenate)(w53, w45) -> (w51:cluster{"X":dbl, "Y":dbl}[])
    "XY Graph 3" <- w51
    n22 = Wait (ms)(milliseconds to wait="dt 2") -> ()  [unwired: 1 out]
    n23 = call "sub_slope_calculate.vi"("point n+1"=w50, "point n"=w45) -> ("deg_gps-base"=w47:dbl)  [unwired: 7 in, 2 out]
    n24 = call "sub_measure_distance.vi"("pt 2"=w50, "pt 1"=w45) -> ("distance"=w48:dbl)  [unwired: 9 in]
    n25 = Bundle("deg_gps-base"=w47, "distance"=w48) -> (w49:cluster{"deg_gps-base":dbl, "distance":dbl})  [unwired: 1 in]
  }
  n26 = while {
    tunnel: w8 -> [w57]
    stop <- "stop" stop-if-true
    n27 = Index Array(array=w57, index="index") -> (element=w55:cluster{"Array":cluster{"x":dbl, "y":dbl}[]})
    n28 = Unbundle(w55) -> ("Array"=→"XY Graph":cluster{"x":dbl, "y":dbl}[])
    n29 = Wait (ms)(milliseconds to wait=u32 100) -> ()  [unwired: 1 out]
  }
  "XY 그래프" <- w7
